vi "StickEncoder.vi"(8 "error in (no error)":errorcluster, 11 "Reset Counter":bool) -> (0 "error out":errorcluster, 3 "PresentPOS(deg)":dbl)   [LabVIEW 2019, in "MotorPID.lvlib"]
uses:
  MotorPID.lvlib
  KNRm_ReMi_OS5.lvlibp/KNRm_ReMi_Toolkit/IO/LowLevel/IO_Channel_Motor.ctl
  KNRm_ReMi_OS5.lvlibp
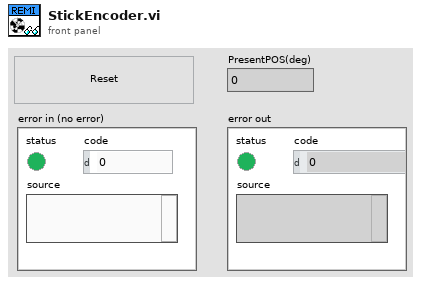
[diagram p1: front panel]
types:
  T1 = typedef "KNRm_ReMi_OS5.lvlibp/IO_Channel_Motor.ctl" = enum16{"M1", "M2", "M3", "M4"}
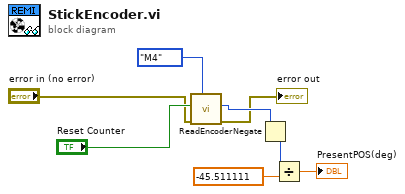
[diagram p0: block diagram]
diagram:
  n1 = call "ReadEncoder.vi"("Channel"=IO_Channel_Motor."M4", "error in"="error in (no error)", "Reset"="Reset Counter") -> ("error out"=→"error out":errorcluster, "ENC (count)"=w3:i32)  [unwired: 7 in]
  n2 = Negate(x=w3) -> (-x=w1:i32)
  n3 = Divide(x=w1, y=-45.511111) -> (x/y=→"PresentPOS(deg)":dbl)
